vi "Write Column 3 to Table.vi"(0 "2D Array In":dbl[][](array[numeric]), 5 "Column 3":dbl[](array[numeric])) -> (4 "2D Array Out":dbl[][](array[numeric]))   [LabVIEW 2010]
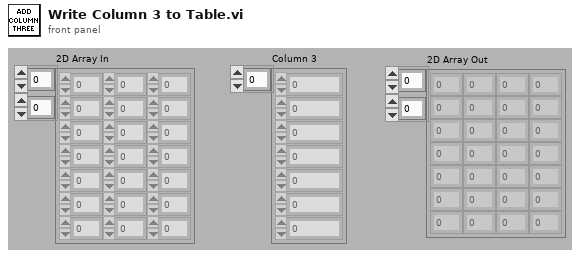
[diagram p1: front panel]
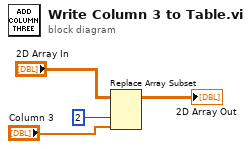
[diagram p0: block diagram]
diagram:
  n1 = Replace Array Subset(array="2D Array In", new element="Column 3", index (col)=2 ("disabled index (col)")) -> (→"2D Array Out":dbl[][])  [unwired: 1 in]
